vi "Set Mag str (SubVI).vi"(10 "字符串":string, 11 ".NET引用句柄输入":refnum<k24>) -> (0 "错误输出":errorcluster)   [LabVIEW 2019, in "Take Seq.lvlib"]
uses:
  Take Seq.lvlib
  lib/QDInstrument.dll
  SubVI.lvlib
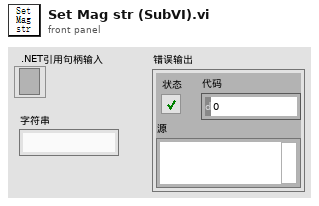
[diagram p1: front panel]
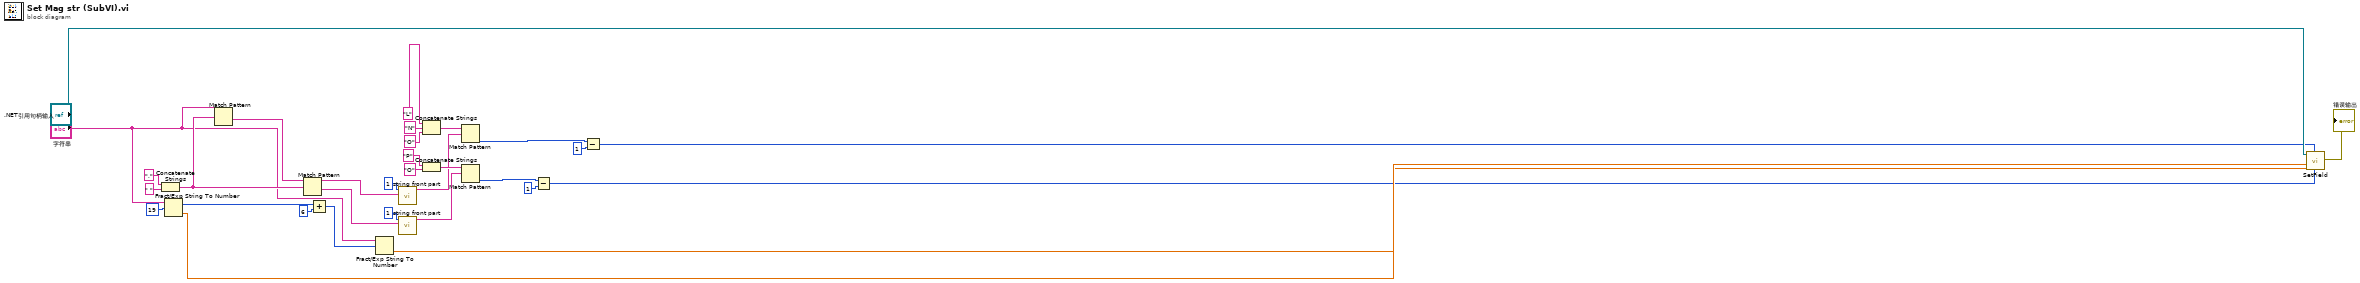
[diagram p0: block diagram]
diagram:
  n1 = Concatenate Strings("," ("字符串"), " " ("字符串")) -> (w29:string)
  n2 = Fract/Exp String To Number(string="字符串", offset=19 ("偏移量")) -> (offset past number=w3:i32, number=w32:dbl)  [unwired: 2 in]
  n3 = Match Pattern(string="字符串", regular expression=w29) -> (after substring=w1:string)  [unwired: 1 in, 3 out]
  n4 = Match Pattern(string=w1, regular expression=w29) -> (before substring=w22:string, after substring=w23:string)  [unwired: 1 in, 2 out]
  n5 = Add(x=w3, y=6) -> (x+y=w4:i32)
  n6 = Fract/Exp String To Number(string="字符串", offset=w4) -> (number=w6:dbl)  [unwired: 2 in, 1 out]
  n7 = call "string front part.vi"("字符串"=w22, "偏移量(0)"=1) -> ("result string"=w9:string)  [unwired: 9 in]
  n8 = call "string front part.vi"("字符串"=w23, "偏移量(0)"=1) -> ("result string"=w17:string)  [unwired: 9 in]
  n9 = Concatenate Strings("L" ("字符串"), "N" ("字符串"), "O" ("字符串")) -> (w13:string)
  n10 = Concatenate Strings("P" ("字符串"), "O" ("字符串")) -> (w20:string)
  n11 = Match Pattern(string=w13, regular expression=w9) -> (offset past match=w14:i32)  [unwired: 1 in, 3 out]
  n12 = Match Pattern(string=w20, regular expression=w17) -> (offset past match=w21:i32)  [unwired: 1 in, 3 out]
  n13 = Subtract(x=w21, y=1) -> (x-y=w25:i32)
  n14 = Subtract(x=w14, y=1) -> (x-y=w26:i32)
  n15 = call "SetField.vi"("Mode"=w25, "Approach"=w26, "Rate"=w6, "Field"=w32, "Instrument Ref In"=".NET引用句柄输入") -> ("error out"=→"错误输出":errorcluster)  [unwired: 2 in, 2 out]
